vi "Werte ändern (Int32_8xZ.I._Rechteck) (SubVI).vi"(0 "geladene Werte (Zeit (s); Wert)":dbl[][](array[numeric]), 1 "Zykluslänge":dbl, 2 "Z.I.":string, 3 "Info":string, 4 "Format+Namen":string) -> (5 "Ausgang":dbl[][](array[numeric]) format="%.2f", 6 "Z.I.":string, 7 "Sperre":bool)   [LabVIEW 2010]
panel:
  out "Fehlermeldung":string="Zeit ist größer als Zykluslänge"
  in  "löschen":bool
  in  "Werte":i32[](array[numeric])
  in  "Zeit (s)":dbl[](array[numeric])
  out "aktuel 8":dbl
  out "aktuel 7":dbl
  out "aktuel 6":dbl
  out "aktuel 5":dbl
  out "aktuel 4":dbl
  out "aktuel 3":dbl
  out "aktuel2":dbl
  out "Name 8":string
  in  "Numerisch 8":dbl
  out "Name 7":string
  in  "Numerisch 7":dbl
  out "Name 6":string
  in  "Numerisch 6":dbl
  out "Name 5":string
  in  "Numerisch 5":dbl
  out "Name 4":string
  in  "Numerisch 4":dbl
  out "Name 3":string
  in  "Numerisch 3":dbl
  out "Name 2":string
  in  "Numerisch 2":dbl
  out "aktuel1":dbl
  out "Name 1":string
  in  "Numerisch 1":dbl
  out "aktuell (Zeit (s); Wert)":dbl[][](array[numeric])
  out "XY Graph":cluster{dbl[], dbl[]}[](graph) caption="XY-Graph"
  out "Zykluslänge":dbl format="%.2f"
  out "Info":string
  in  "ändern":bool
  in  "Stopp":bool
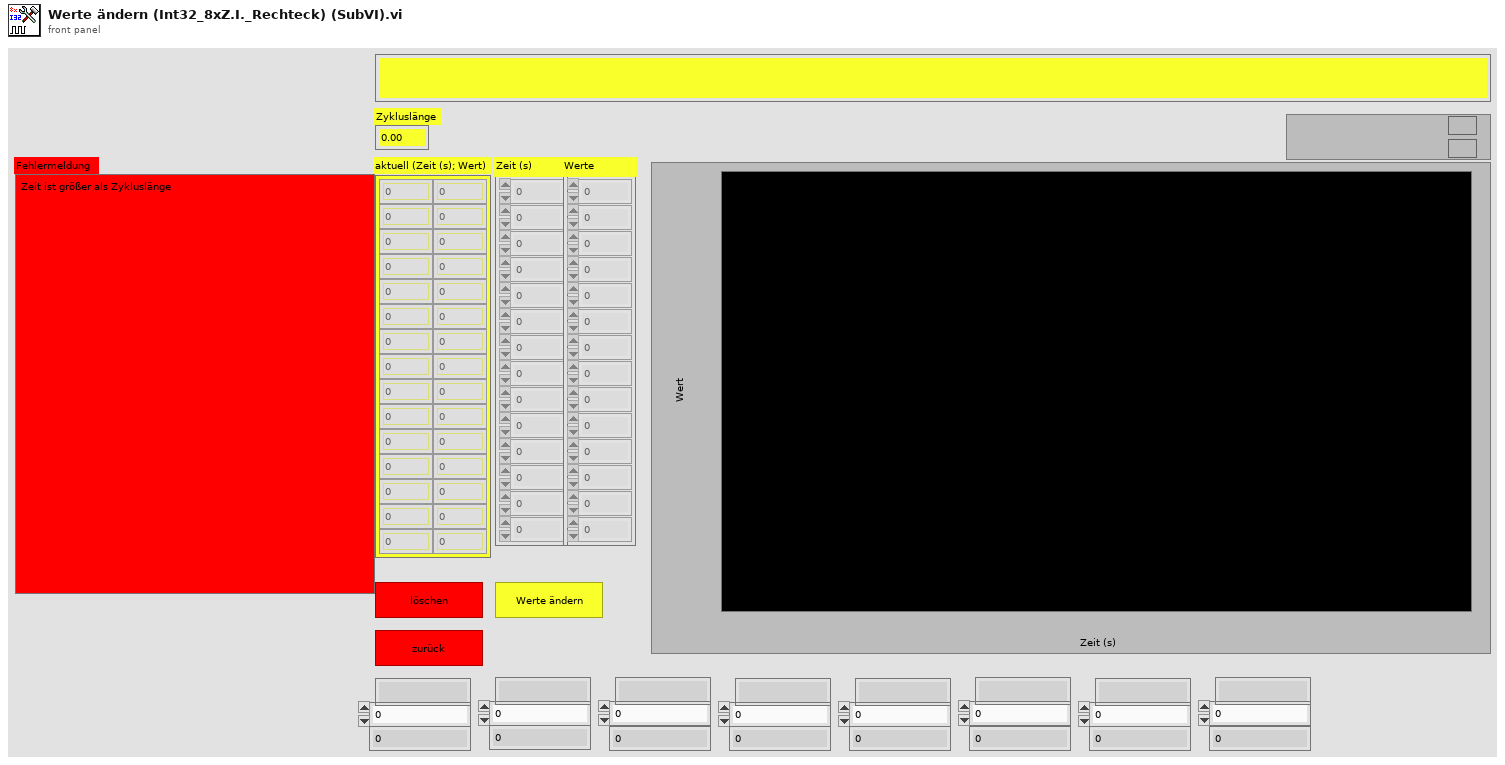
[diagram p1: front panel]
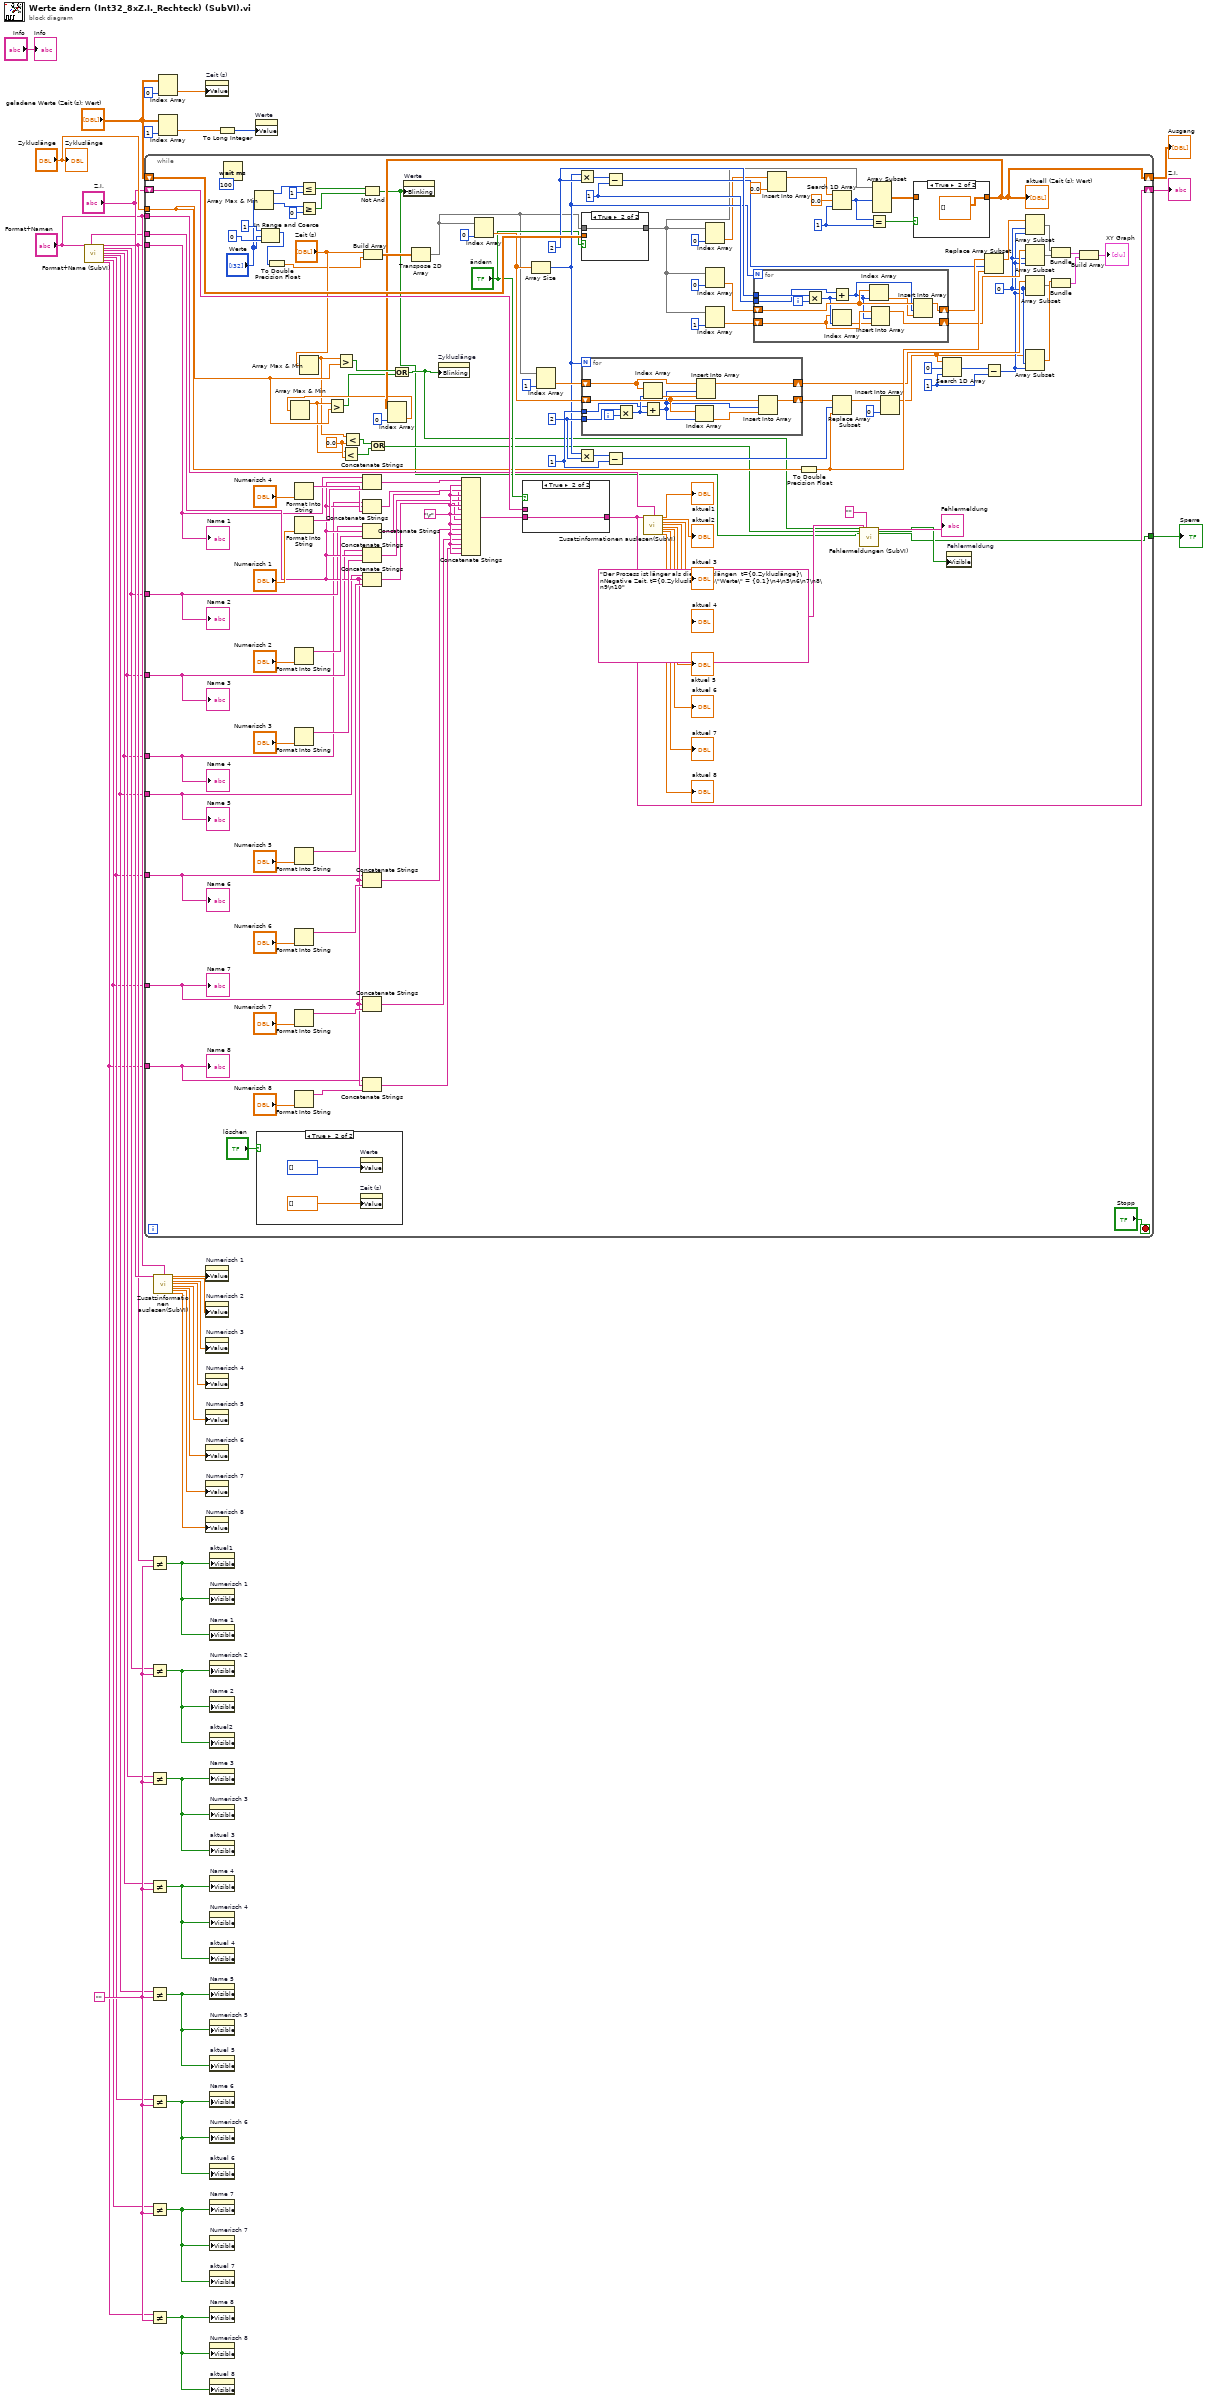
[diagram p0: block diagram]
diagram:
  w18 = ""
  n1 = call "Format+Name (SubVI).vi"("Format+Namen Eingang"="Format+Namen") -> ("Trennzeichen"=w10:string, "1"=w9:string, "2"=w8:string, "3"=w7:string, "4"=w6:string, "5"=w5:string, "6"=w4:string, "7"=w3:string, "8"=w2:string)  [unwired: 15 in, 3 out]
  n2 = while {
    shift-right: [w60] -> w39
    shift-left: "geladene Werte (Zeit (s); Wert)" -> [w169]
    tunnel: "Zykluslänge" -> [w62]
    shift-right: [w115] -> w36
    shift-left: "Z.I." -> [w120]
    tunnel: w9 -> [w75]
    tunnel: w10 -> [w99]
    tunnel: "Format+Namen" -> [w65]
    tunnel: w8 -> [w89]
    tunnel: w7 -> [w88]
    tunnel: w6 -> [w76]
    tunnel: w5 -> [w87]
    tunnel: w4 -> [w86]
    tunnel: w3 -> [w85]
    tunnel: w2 -> [w84]
    tunnel: [w50] -> w1
    stop <- "Stopp" stop-if-true
    w45 = 0.0 ("y")
    w98 = "\r"
    w123 = 1 ("Deaktivierter Index (Zeile)")
    w137 = 0 ("Index")
    w143 = 1 ("Startindex (0)")
    w155 = 1 ("y")
    w154 = 2 ("y")
    w161 = 1 ("y")
    w157 = 2 ("y")
    n3 = Wait (ms)(milliseconds to wait=u32 100 ("Zu wartende ms")) -> ()  [unwired: 1 out]
    n4 = Array Max & Min(array="Werte") -> (max value=w74:i32, min value=w72:i32)  [unwired: 2 out]
    n5 = case shown="True" "löschen" {
      frame False {
      }
      frame True {
        n6 = property on="Werte" class="Arr (strikt)"("Value"=i32[] []) -> ()  [unwired: 2 in, 2 out]
        n7 = property on="Zeit (s)" class="Arr (strikt)"("Value"=dbl[] []) -> ()  [unwired: 2 in, 2 out]
      }
    }
    n8 = In Range and Coerce(upper limit=1 ("y"), x="Werte", lower limit=0 ("y")) -> (coerced(x)=w54:i32[])  [unwired: 1 out]
    n9 = To Double Precision Float(number=w54) -> (double precision float=w53:dbl[])
    n10 = Format Into String("Numerisch 4") -> (resulting string=w109:string)  [unwired: 3 in, 1 out]
    n11 = Format Into String("Numerisch 1") -> (resulting string=w117:string)  [unwired: 3 in, 1 out]
    n12 = Format Into String("Numerisch 2") -> (resulting string=w113:string)  [unwired: 3 in, 1 out]
    n13 = Format Into String("Numerisch 3") -> (resulting string=w110:string)  [unwired: 3 in, 1 out]
    n14 = Format Into String("Numerisch 5") -> (resulting string=w106:string)  [unwired: 3 in, 1 out]
    n15 = Format Into String("Numerisch 6") -> (resulting string=w105:string)  [unwired: 3 in, 1 out]
    n16 = Format Into String("Numerisch 7") -> (resulting string=w102:string)  [unwired: 3 in, 1 out]
    n17 = Format Into String("Numerisch 8") -> (resulting string=w101:string)  [unwired: 3 in, 1 out]
    n18 = Less Or Equal?(x=w74, y=1) -> (x <= y?=w70:bool)
    n19 = Greater Or Equal?(x=w72, y=0) -> (x >= y?=w69:bool)
    n20 = Array Max & Min(array="Zeit (s)") -> (max value=w43:dbl)  [unwired: 3 out]
    n21 = Greater?(x=w43, y=w62) -> (0:w63:bool)
    n22 = Less?(x=w43, y=w45) -> (x < y?=w47:bool)
    n23 = Concatenate Strings(w75, w99, w117) -> (w97:string)
    n24 = Concatenate Strings(w76, w99, w109) -> (w94:string)
    n25 = Concatenate Strings(w89, w99, w113) -> (w96:string)
    n26 = Concatenate Strings(w88, w99, w110) -> (w95:string)
    n27 = Concatenate Strings(w87, w99, w106) -> (w93:string)
    n28 = Concatenate Strings(w86, w99, w105) -> (w92:string)
    n29 = Concatenate Strings(w85, w99, w102) -> (w91:string)
    n30 = Concatenate Strings(w84, w99, w101) -> (w90:string)
    n31 = Not And(1:w69, 2:w70) -> (0:w41:bool)
    n32 = Build Array("Zeit (s)", w53) -> (w68:dbl[][])
    n33 = property on="Werte" class="Arr (strikt)"("Blinking"=w41) -> ()  [unwired: 2 in, 2 out]
    n34 = Transpose 2D Array(2D array=w68) -> (transposed array=w67:dbl[][])
    n35 = Concatenate Strings(w97, w98, w96, w98, w95, w98, w94, w98, w93, w98, w92, w98, w91, w98, w90, w98) -> (w116:string)
    n36 = Index Array(array=w67, index (col)=0 ("Deaktivierter Index (Spalte)")) -> (element=w164:dbl[])  [unwired: 1 in]
    n37 = case shown="True" "ändern" {
      tunnel: w120 -> [w174 _]
      tunnel: [w174 w175] -> w115
      tunnel: w116 -> [_ w175]
      frame False {
      }
      frame True {
      }
    }
    n38 = Array Size(array=w164) -> (size(s)=w147:i32)
    n39 = Index Array(array=w67, index (col)=1 ("Deaktivierter Index (Spalte)")) -> (element=w163:dbl[])  [unwired: 1 in]
    n40 = Multiply(x=w147, y=w154) -> (x*y=w156:i32)
    n41 = Multiply(x=w147, y=w157) -> (x*y=w162:i32)
    n42 = case shown="True" "ändern" {
      tunnel: w169 -> [w200 _]
      tunnel: [w200 w201] -> w125
      tunnel: w67 -> [_ w201]
      frame False {
      }
      frame True {
      }
    }
    n43 = for {
      N: w147 -> [_]
      shift-right: [w198] -> w145
      shift-left: w164 -> [w197]
      shift-right: [w193] -> w141
      shift-left: w163 -> [w195]
      tunnel: w157 -> [w190]
      tunnel: w161 -> [w189]
      i -> [w199]
      n44 = Multiply(x=w190, y=w199) -> (x*y=w196:i32)
      n45 = Index Array(array=w195, index=w196) -> (element=w194:dbl)
      n46 = Add(x=w189, y=w196) -> (x+y=w191:i32)
      n47 = Index Array(array=w197, index=w191) -> (element=w192:dbl)
      n48 = Insert Into Array(array=w195, index=w191, new element=w194) -> (w193:dbl[])
      n49 = Insert Into Array(array=w197, index=w191, new element=w192) -> (w198:dbl[])
    }
    n50 = Subtract(x=w156, y=w155) -> (x-y=w152:i32)
    n51 = Subtract(x=w162, y=w161) -> (x-y=w160:i32)
    n52 = call "Zusatzinformationen auslesen(SubVI).vi"("Zusatzinformationen"=w115, "Format+Namen"=w65) -> ("1"=→"aktuel1":dbl, "2"=→"aktuel2":dbl, "3"=→"aktuel 3":dbl, "4"=→"aktuel 4":dbl, "5"=→"aktuel 5":dbl, "6"=→"aktuel 6":dbl, "7"=→"aktuel 7":dbl, "8"=→"aktuel 8":dbl)  [unwired: 18 in]
    n53 = Index Array(array=w125, index (col)=0 ("Deaktivierter Index (Spalte)")) -> (element=w127:dbl[])  [unwired: 1 in]
    n54 = Index Array(array=w125, index (col)=0 ("Deaktivierter Index (Spalte)")) -> (element=w149:dbl[])  [unwired: 1 in]
    n55 = Index Array(array=w125, index (col)=1 ("Deaktivierter Index (Spalte)")) -> (element=w148:dbl[])  [unwired: 1 in]
    n56 = for {
      N: w147 -> [_]
      shift-right: [w187] -> w153
      shift-left: w149 -> [w186]
      shift-right: [w182] -> w139
      shift-left: w148 -> [w184]
      tunnel: w154 -> [w179]
      tunnel: w155 -> [w178]
      i -> [w188]
      n57 = Multiply(x=w179, y=w188) -> (x*y=w185:i32)
      n58 = Add(x=w178, y=w185) -> (x+y=w180:i32)
      n59 = Index Array(array=w184, index=w185) -> (element=w183:dbl)
      n60 = Index Array(array=w186, index=w180) -> (element=w181:dbl)
      n61 = Insert Into Array(array=w184, index=w180, new element=w183) -> (w182:dbl[])
      n62 = Insert Into Array(array=w186, index=w180, new element=w181) -> (w187:dbl[])
    }
    n63 = Insert Into Array(array=w127, new element=0.0 ("Neues Element/Teil-Array")) -> (w126:dbl[])  [unwired: 1 in]
    n64 = To Double Precision Float(number=w62) -> (double precision float=w151:dbl)
    n65 = Search 1D Array(1D array=w126, element=0.0 ("Element"), start index (0)=w123) -> (index of element=w124:i32)
    n66 = Replace Array Subset(array=w145, new element=w151, index=w160) -> (w133:dbl[])
    n67 = Equal?(x=w124, y=w123) -> (x = y?=w122:bool)
    n68 = Array Subset(array=w125, length (row)=w124) -> (w121:dbl[][])  [unwired: 3 in]
    n69 = Insert Into Array(array=w133, new element=0 ("Neues Element/Teil-Array")) -> (w132:dbl[])  [unwired: 1 in]
    n70 = case shown="True" w122 {
      tunnel: w121 -> [w176 _]
      tunnel: [w176 dbl[][] [] ("neue Werte (Zeit (s); Wert)")] -> w60
      frame False {
      }
      frame True {
      }
    }
    "aktuell (Zeit (s); Wert)" <- w60
    n71 = Index Array(array=w60, index (col)=0 ("Deaktivierter Index (Spalte)")) -> (element=w59:dbl[])  [unwired: 1 in]
    n72 = Array Max & Min(array=w59) -> (max value=w44:dbl)  [unwired: 3 out]
    n73 = Greater?(x=w44, y=w62) -> (0:w58:bool)
    n74 = Less?(x=w44, y=w45) -> (x < y?=w46:bool)
    n75 = Or(x=w47, y=w46) -> (x .or. y?=w42:bool)
    n76 = Or(x=w63, y=w58) -> (x .or. y?=w48:bool)
    n77 = property on="Zykluslänge" class="DigWert (strikt)"("Blinking"=w48) -> ()  [unwired: 2 in, 2 out]
    n78 = call "Fehlermeldungen (SubVI).vi"("Fehler 1"=w48, "Fehler 2"=w42, "Fehler 3"=w41, "Fehlermeldungen Namen"="Der Prozess ist länger als die Zykluslängen  t={0,Zykluslänge}\nNegative Zeit. t={0,Zykluslänge}\n\"Werte\" = {0,1}\n4\n5\n6\n7\n8\n9\n10", "Kritischefehler Positionen"="") -> ("Fehlermeldung Ausgang"=→"Fehlermeldung":string, "Fehler?"=w51:bool, "Sperre"=w50:bool)  [unwired: 20 in]
    n79 = Search 1D Array(1D array=w132, element=0 ("Element"), start index (0)=w143) -> (index of element=w144:i32)
    n80 = property on="Fehlermeldung" class="Str"("Visible"=w51) -> ()  [unwired: 2 in, 2 out]
    n81 = Replace Array Subset(array=w153, new element=w151, index=w152) -> (w135:dbl[])
    n82 = Subtract(x=w144, y=w143) -> (x-y=w136:i32)
    n83 = Array Subset(array=w135, index=w137, length=w136) -> (w134:dbl[])
    n84 = Array Subset(array=w139, index=w137, length=w136) -> (w138:dbl[])
    n85 = Array Subset(array=w141, index=w137, length=w136) -> (w140:dbl[])
    n86 = Array Subset(array=w132, index=w137, length=w136) -> (w142:dbl[])
    n87 = Bundle(w134, w138) -> (w150:cluster{dbl[], dbl[]})  [unwired: 1 in]
    n88 = Bundle(w142, w140) -> (w158:cluster{dbl[], dbl[]})  [unwired: 1 in]
    n89 = Build Array(w150, w158) -> (→"XY Graph":cluster{dbl[], dbl[]}[])
    "Name 1" <- w75
    "Name 2" <- w89
    "Name 3" <- w88
    "Name 4" <- w76
    "Name 5" <- w87
    "Name 6" <- w86
    "Name 7" <- w85
    "Name 8" <- w84
  }
  "Ausgang" <- w39
  "Z.I." <- w36
  "Sperre" <- w1
  n90 = Not Equal?(x=w9, y=w18) -> (x != y?=w26:bool)
  n91 = Not Equal?(x=w8, y=w18) -> (x != y?=w25:bool)
  n92 = Not Equal?(x=w7, y=w18) -> (x != y?=w24:bool)
  n93 = Not Equal?(x=w6, y=w18) -> (x != y?=w23:bool)
  n94 = Not Equal?(x=w5, y=w18) -> (x != y?=w22:bool)
  n95 = Not Equal?(x=w4, y=w18) -> (x != y?=w21:bool)
  n96 = Not Equal?(x=w3, y=w18) -> (x != y?=w20:bool)
  n97 = Not Equal?(x=w2, y=w18) -> (x != y?=w19:bool)
  n98 = call "Zusatzinformationen auslesen(SubVI).vi"("Zusatzinformationen"="Z.I.", "Format+Namen"="Format+Namen") -> ("1"=w34:dbl, "2"=w33:dbl, "3"=w32:dbl, "4"=w31:dbl, "5"=w30:dbl, "6"=w29:dbl, "7"=w28:dbl, "8"=w27:dbl)  [unwired: 18 in]
  n99 = Index Array(array="geladene Werte (Zeit (s); Wert)", index (col)=0 ("Deaktivierter Index (Spalte)")) -> (element=w14:dbl[])  [unwired: 1 in]
  n100 = Index Array(array="geladene Werte (Zeit (s); Wert)", index (col)=1 ("Deaktivierter Index (Spalte)")) -> (element=w13:dbl[])  [unwired: 1 in]
  n101 = property on="Zeit (s)" class="Arr (strikt)"("Value"=w14) -> ()  [unwired: 2 in, 2 out]
  n102 = property on="Numerisch 1" class="DigWert (strikt)"("Value"=w34) -> ()  [unwired: 2 in, 2 out]
  n103 = property on="Numerisch 2" class="DigWert (strikt)"("Value"=w33) -> ()  [unwired: 2 in, 2 out]
  n104 = property on="Numerisch 3" class="DigWert (strikt)"("Value"=w32) -> ()  [unwired: 2 in, 2 out]
  n105 = property on="Numerisch 4" class="DigWert (strikt)"("Value"=w31) -> ()  [unwired: 2 in, 2 out]
  n106 = property on="Numerisch 5" class="DigWert (strikt)"("Value"=w30) -> ()  [unwired: 2 in, 2 out]
  n107 = property on="Numerisch 6" class="DigWert (strikt)"("Value"=w29) -> ()  [unwired: 2 in, 2 out]
  n108 = property on="Numerisch 7" class="DigWert (strikt)"("Value"=w28) -> ()  [unwired: 2 in, 2 out]
  n109 = property on="Numerisch 8" class="DigWert (strikt)"("Value"=w27) -> ()  [unwired: 2 in, 2 out]
  n110 = property on="aktuel1" class="DigWert (strikt)"("Visible"=w26) -> ()  [unwired: 2 in, 2 out]
  n111 = property on="Numerisch 1" class="DigWert (strikt)"("Visible"=w26) -> ()  [unwired: 2 in, 2 out]
  n112 = property on="Name 1" class="Str"("Visible"=w26) -> ()  [unwired: 2 in, 2 out]
  n113 = property on="Numerisch 2" class="DigWert (strikt)"("Visible"=w25) -> ()  [unwired: 2 in, 2 out]
  n114 = property on="Name 2" class="Str"("Visible"=w25) -> ()  [unwired: 2 in, 2 out]
  n115 = property on="aktuel2" class="DigWert (strikt)"("Visible"=w25) -> ()  [unwired: 2 in, 2 out]
  n116 = property on="Name 3" class="Str"("Visible"=w24) -> ()  [unwired: 2 in, 2 out]
  n117 = property on="Numerisch 3" class="DigWert (strikt)"("Visible"=w24) -> ()  [unwired: 2 in, 2 out]
  n118 = property on="aktuel 3" class="DigWert (strikt)"("Visible"=w24) -> ()  [unwired: 2 in, 2 out]
  n119 = property on="Name 4" class="Str"("Visible"=w23) -> ()  [unwired: 2 in, 2 out]
  n120 = property on="Numerisch 4" class="DigWert (strikt)"("Visible"=w23) -> ()  [unwired: 2 in, 2 out]
  n121 = property on="aktuel 4" class="DigWert (strikt)"("Visible"=w23) -> ()  [unwired: 2 in, 2 out]
  n122 = property on="Name 5" class="Str"("Visible"=w22) -> ()  [unwired: 2 in, 2 out]
  n123 = property on="Numerisch 5" class="DigWert (strikt)"("Visible"=w22) -> ()  [unwired: 2 in, 2 out]
  n124 = property on="aktuel 5" class="DigWert (strikt)"("Visible"=w22) -> ()  [unwired: 2 in, 2 out]
  n125 = property on="Name 6" class="Str"("Visible"=w21) -> ()  [unwired: 2 in, 2 out]
  n126 = property on="Numerisch 6" class="DigWert (strikt)"("Visible"=w21) -> ()  [unwired: 2 in, 2 out]
  n127 = property on="aktuel 6" class="DigWert (strikt)"("Visible"=w21) -> ()  [unwired: 2 in, 2 out]
  n128 = property on="Name 7" class="Str"("Visible"=w20) -> ()  [unwired: 2 in, 2 out]
  n129 = property on="Numerisch 7" class="DigWert (strikt)"("Visible"=w20) -> ()  [unwired: 2 in, 2 out]
  n130 = property on="aktuel 7" class="DigWert (strikt)"("Visible"=w20) -> ()  [unwired: 2 in, 2 out]
  n131 = property on="Name 8" class="Str"("Visible"=w19) -> ()  [unwired: 2 in, 2 out]
  n132 = property on="Numerisch 8" class="DigWert (strikt)"("Visible"=w19) -> ()  [unwired: 2 in, 2 out]
  n133 = property on="aktuel 8" class="DigWert (strikt)"("Visible"=w19) -> ()  [unwired: 2 in, 2 out]
  n134 = To Long Integer(number=w13) -> (32bit integer=w12:i32[])
  n135 = property on="Werte" class="Arr (strikt)"("Value"=w12) -> ()  [unwired: 2 in, 2 out]
  "Info" <- "Info"
  "Zykluslänge" <- "Zykluslänge"
